vi "Sets the Reference Value for the Percent Function.vi"(5 "Enable to Query":bool=TRUE, 7 "Enable to Sets":bool=TRUE, 8 "error in":errorcluster, 10 "Reference Value for Percent":dbl format="%#.6g", 11 "VISA resource name":refnum<visa-resource-name>) -> (0 "error out":errorcluster, 2 "Return the Reference Value":string, 3 "VISA resource name out":refnum<visa-resource-name>)   [LabVIEW 2011, in "DMM4.lvlib"]
uses:
  <instrlib>/DMM4/DMM4.lvlib
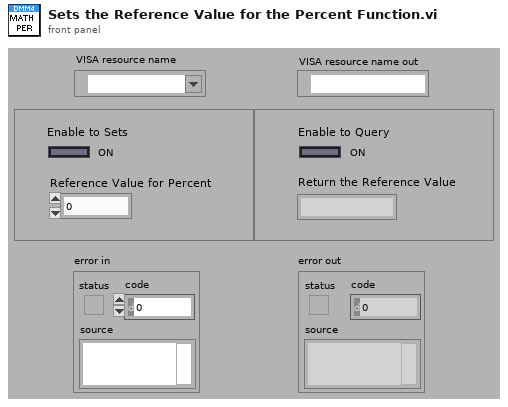
[diagram p1: front panel]
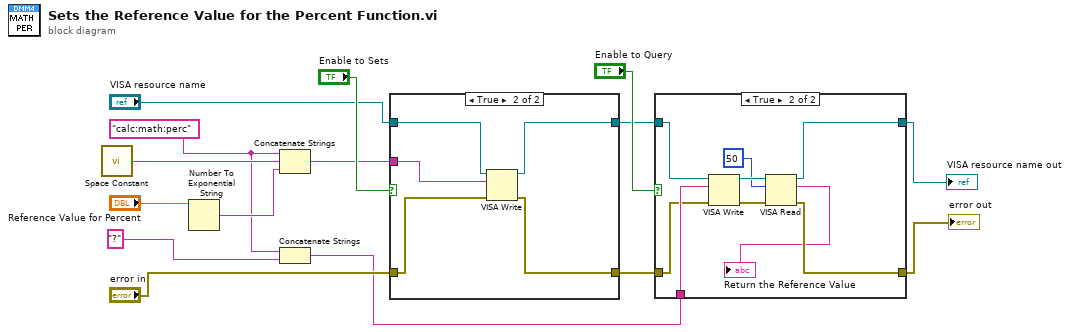
[diagram p0: block diagram]
diagram:
  w13 = "calc:math:perc"
  n1 = call <vilib>:"Space Constant.vi"() -> ("String"=w15:string)
  n2 = Number To Exponential String(number="Reference Value for Percent") -> (E-format string=w14:string)  [unwired: 3 in]
  n3 = Concatenate Strings(w13, w15, w14) -> (w10:string)
  n4 = Concatenate Strings(w13, "?") -> (w4:string)
  n5 = case shown="True" "Enable to Sets" {
    tunnel: w10 -> [_ w22]
    tunnel: "VISA resource name" -> [w17 w21]
    tunnel: "error in" -> [w16 w20]
    tunnel: [w17 w19] -> w6
    tunnel: [w16 w18] -> w5
    frame False {
    }
    frame True {
      n6 = VISA Write(VISA resource name=w21, write buffer=w22, error in (no error)=w20) -> (VISA resource name out=w19:refnum<visa-resource-name>, error out=w18:errorcluster)  [unwired: 1 out]
    }
  }
  n7 = case shown="True" "Enable to Query" {
    tunnel: w6 -> [w24 w29]
    tunnel: w5 -> [w23 w28]
    tunnel: [w24 w27] -> w3
    tunnel: [w23 w26] -> w2
    tunnel: w4 -> [_ w30]
    frame False {
    }
    frame True {
      n8 = VISA Write(VISA resource name=w29, write buffer=w30, error in (no error)=w28) -> (VISA resource name out=w32:refnum<visa-resource-name>, error out=w33:errorcluster)  [unwired: 1 out]
      n9 = VISA Read(VISA resource name=w32, byte count=u32 50, error in (no error)=w33) -> (VISA resource name out=w27:refnum<visa-resource-name>, read buffer=→"Return the Reference Value":string, error out=w26:errorcluster)  [unwired: 1 out]
    }
  }
  "VISA resource name out" <- w3
  "error out" <- w2
